vi "Log.vi"(8 "error in (no error)":errorcluster, 10 "Log Text":string, 11 "Custom Sink in":refnum<class "Custom Sink.lvclass">) -> (0 "error out":errorcluster, 3 "Custom Sink out":refnum<class "Custom Sink.lvclass">)   [LabVIEW 2020, in "Custom Sink.lvclass"]
uses:
  Custom Sink.lvclass
  Custom Sink.lvclass/Custom Sink.ctl
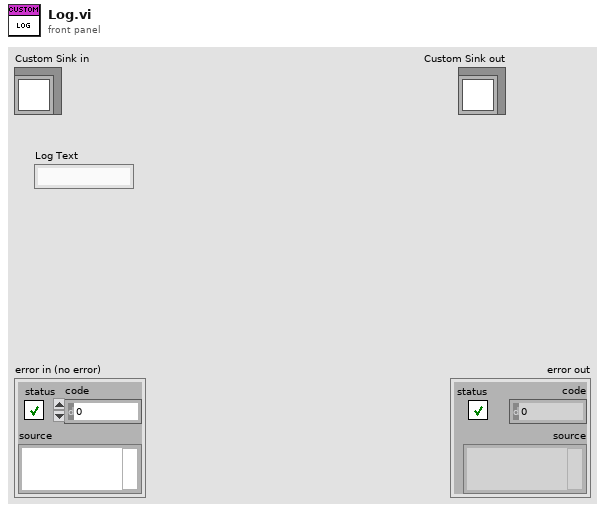
[diagram p1: front panel]
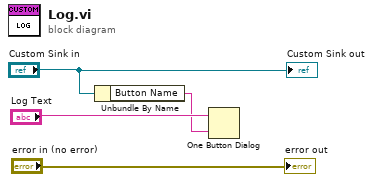
[diagram p0: block diagram]
diagram:
  n1 = Unbundle By Name("Custom Sink in") -> ("Button Name"=w1:string)
  n2 = One Button Dialog(message="Log Text", button name ("OK")=w1) -> ()  [unwired: 1 out]
  "error out" <- "error in (no error)"
  "Custom Sink out" <- "Custom Sink in"
